vi "完数.vi"(1 "范围":i32) -> (0 "完数":i32[](array[numeric]))   [LabVIEW 2012]
doc: "功能：\n\n求三位数中的水仙花数\n\n水仙花数的定义：\n\n所谓水仙花数，是指一个三位数，其各个位数的立方和等于该数本身，比如：\n\n153=1^3+5^+3^\n\ncsxcs_366创建"
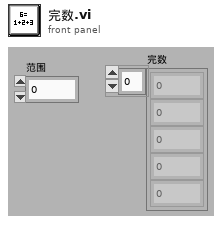
[diagram p1: front panel]
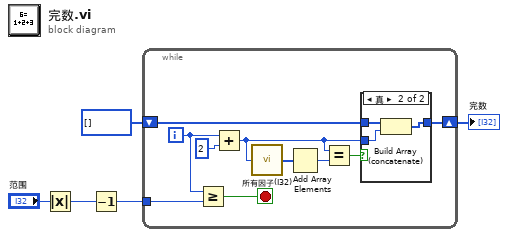
[diagram p0: block diagram]
diagram:
  n1 = Absolute Value(x="范围") -> (abs(x)=w3:i32)
  n2 = Decrement(x=w3) -> (x-1=w4:i32)
  n3 = while {
    tunnel: w4 -> [w15]
    shift-right: [w6] -> w1
    shift-left: i32[] [] -> [w7]
    i -> [w12]
    stop <- w14 stop-if-true
    n4 = Greater Or Equal?(x=w12, y=w15) -> (x >= y?=w14:bool)
    n5 = Add(x=w12, y=2) -> (x+y=w8:i32)
    n6 = call "所有因子(I32).vi"("范围"=w8) -> ("所有因子"=w13:i32[])
    n7 = Add Array Elements(numeric array=w13) -> (sum=w10:i32)
    n8 = Equal?(x=w8, y=w10) -> (x = y?=w9:bool)
    n9 = case shown="真" w9 {
      tunnel: w7 -> [w16 w19]
      tunnel: [w16 w17] -> w6
      tunnel: w8 -> [_ w18]
      frame False {
      }
      frame True {
        n10 = Build Array (concatenate)(w19, w18) -> (w17:i32[])
      }
    }
  }
  "完数" <- w1
